vi "Concatenate_Blocks.vi"() -> (5 "Plug in titles":string[](array[string]), 7 "Plug in values":string[](array[string]))   [LabVIEW 2010]
uses:
  Controls/Instrument_Array.ctl
  Controls/Post_Process.ctl
  Controls/Graph_Type.ctl
  Globals/Meas_global.vi
  Acquisition/PWA/PWAtasksGLOBAL.vi
  Globals/Plug_in_data_global.vi
  <vilib>/Analysis/NI_AALBase.lvlib
  <vilib>/Analysis/NI_AALPro.lvlib
panel:
  in  "Inst Array":T1
  in  "Show Smooth":bool=TRUE
  in  "Save Spectra?":bool
  in  "Desired number of samples per block":i32=4096
  in  "Calculate Spectra and Histogram?":bool
  out "Spectra":cluster{dbl, dbl, "Spectrum output array":dbl[]}(graph)
  in  "Averaging samples":i32=5 min=1 max=1000
  out "XY Graph":cluster{"Axis":dbl[], "Histogram":i32[]}(graph)
  in  "Specta Index":i32
  out "Waveform Graph":dbl[][](graph)
  in  "Channels to Plot":i32[](array[ring])=[0] items=["FF (C)", "Save Nothing"]
  # "Run this VI to update the channel names"
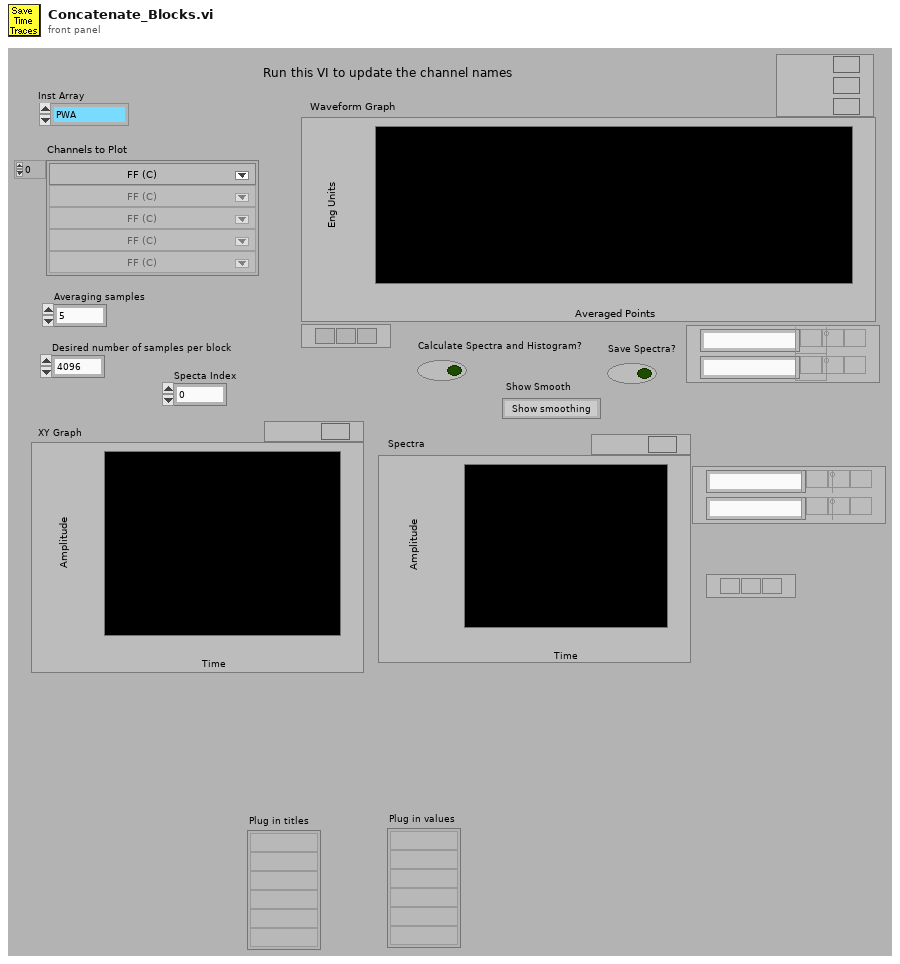
[diagram p1: front panel]
types:
  T1 = typedef "Instrument_Array.ctl" = enum16{"PWA", "LDA", "Analogue"}
  T2 = typedef "Analysis_info_cluster.ctl" = cluster{"Colour":u32, "Inst type":T3, "Inst name":string, "Symbol":string, "Code name":string, "Extra Info":string, "Inst Array":T1, "Index":i32, "Voltage Index":i32, "Extra Titles":string[], "Extra Values":string[]}
  T3 = typedef "Inst_type.ctl" = enum16{"Propeller anemometer", "Raw voltage", "Pressure Transducer", "Pitot-static tube", "Preston tube", "Hot wire", "Cross wire 1", "Cross wire 2", "Generic Linear", "Generic Polynomial", "Generic BackPoly", "Fast FID", "Thermocouple", "Cold wire", "Pulsed Wire", "LDA Vel", "LDA Tran time", "LDA Arr time"}
  T4 = typedef "Post_Process.ctl" = enum16{"Take New Data", "Post Process Raw Data File"}
  T5 = typedef "Graph_Type.ctl" = enum16{"Show no graph", "Voltage trace", "Velocity trace", "Vel histogram", "Spectrum", "f.E(f) v Log f", "Auto-Corr"}
  T6 = cluster{"Plot 1":u16, "Plot 2":u16, "Save graph":u16, "Plot Type":T5}
  T7 = cluster{dbl, dbl, "Spectrum output array":dbl[]}[]
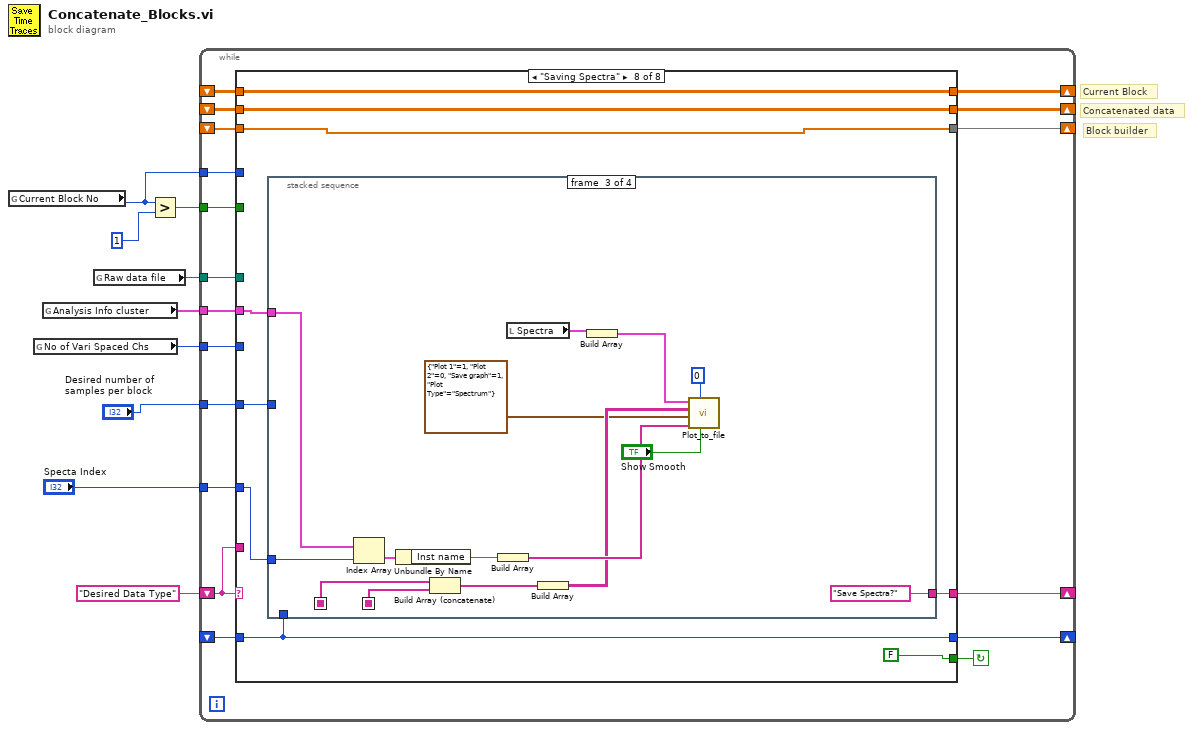
[diagram p0: block diagram]
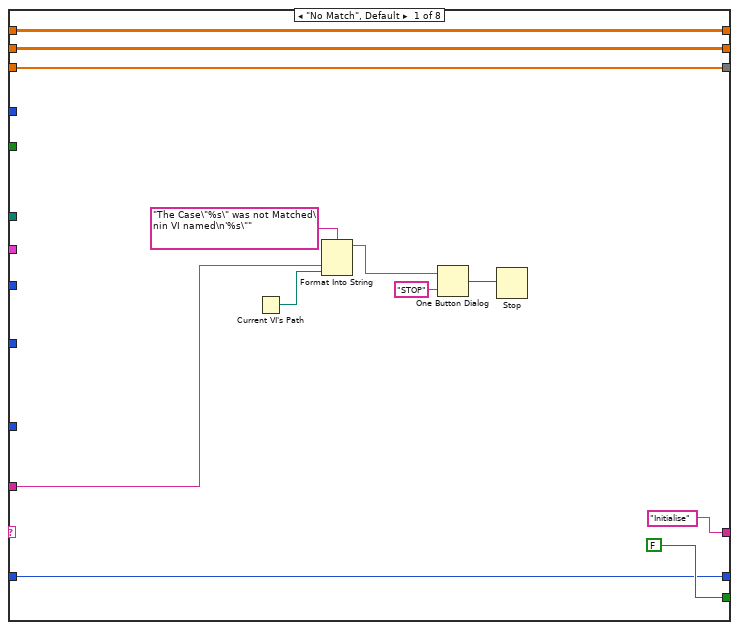
[diagram p2: hidden frame]
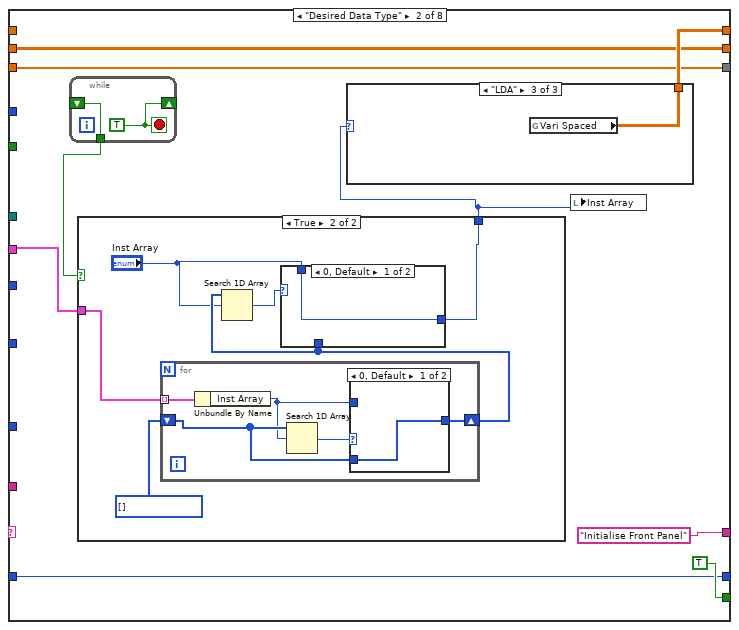
[diagram p3: hidden frame]
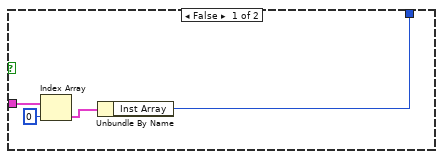
[diagram p4: hidden frame]
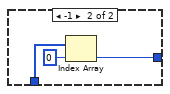
[diagram p5: hidden frame]
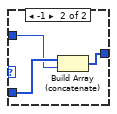
[diagram p6: hidden frame]
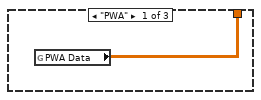
[diagram p7: hidden frame]
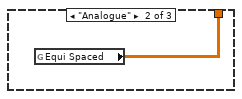
[diagram p8: hidden frame]
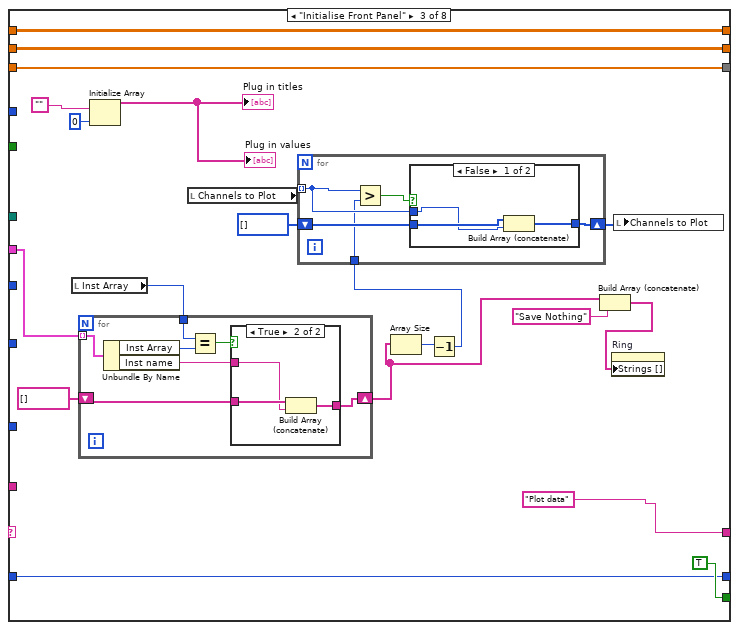
[diagram p9: hidden frame]
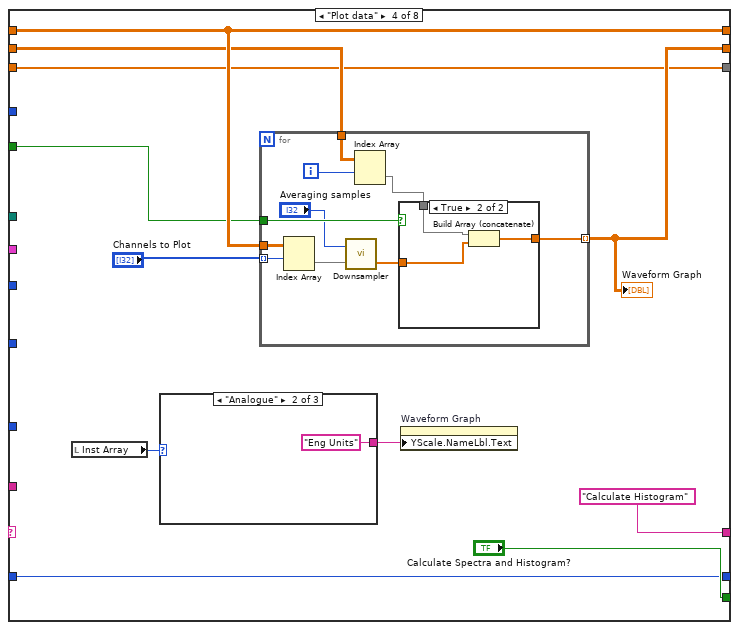
[diagram p12: hidden frame]
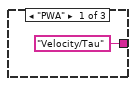
[diagram p13: hidden frame]
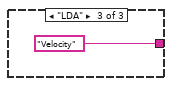
[diagram p14: hidden frame]
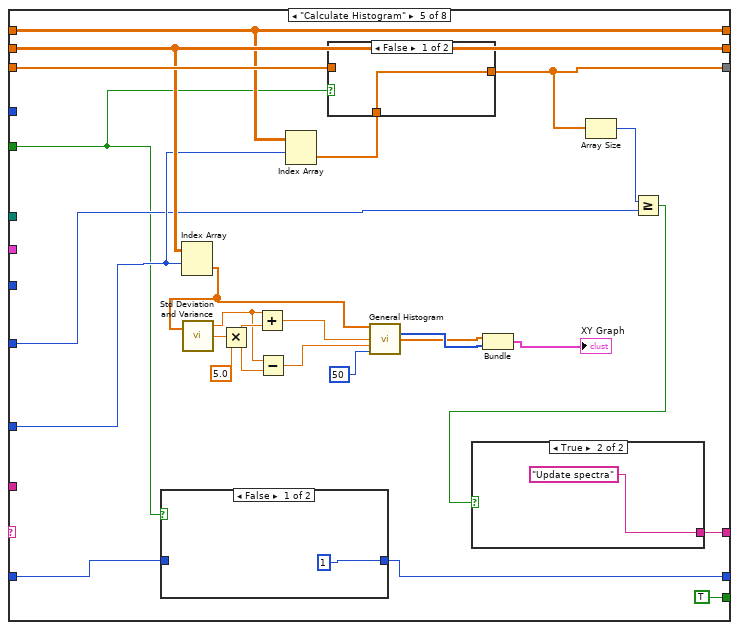
[diagram p16: hidden frame]
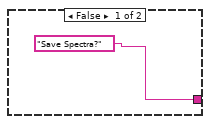
[diagram p18: hidden frame]
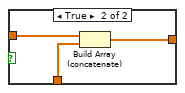
[diagram p19: hidden frame]
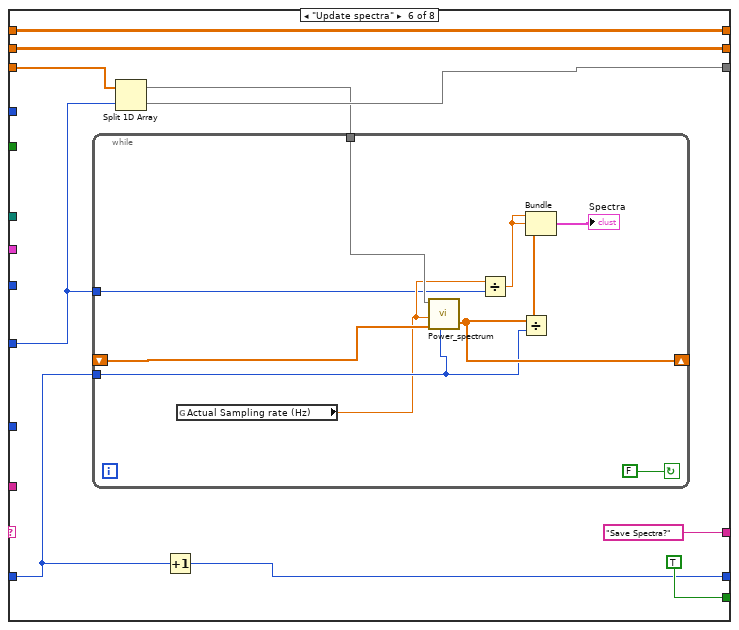
[diagram p20: hidden frame]
diagram:
  # "Block builder"
  # "Concatenated data"
  # "Current Block"
  n1 = global read "Meas_global.vi" "Current Block No"() -> (w6:i32)
  n2 = global read "Meas_global.vi" "No of Vari Spaced Chs"() -> (w4:i32)
  n3 = global read "Meas_global.vi" "Analysis Info cluster"() -> (w5:T2[])
  n4 = global read "Meas_global.vi" "Raw data file"() -> (w8:path)
  n5 = Greater?(x=w6, y=1) -> (0:w3:bool)
  n6 = while {
    shift-left: "Desired Data Type" -> [w25]
    shift-right: [w26] -> _
    tunnel: w8 -> [w24]
    tunnel: w3 -> [w23]
    tunnel: w6 -> [w22]
    tunnel: w5 -> [w21]
    tunnel: w4 -> [w20]
    shift-right: [w19] -> _
    shift-left: _ -> [w18]
    shift-right: [w16] -> _
    shift-left: _ -> [w17]
    shift-right: [w14] -> _
    shift-left: _ -> [w15]
    tunnel: "Desired number of samples per block" -> [w13]
    tunnel: "Specta Index" -> [w12]
    shift-right: [w11] -> _
    shift-left: _ -> [w10]
    stop <- w27 continue-if-true
    n7 = case shown="\"Saving Spectra\"" w25 {
      tunnel: [FALSE TRUE TRUE "Calculate Spectra and Histogram?" TRUE ("Calculate Spectra and Histogram?") TRUE ("Calculate Spectra and Histogram?") w199 FALSE ("Calculate Spectra and Histogram?")] -> w27
      tunnel: ["Initialise" "Initialise Front Panel" "Plot data" "Calculate Histogram" ("t") w149 "Save Spectra?" "Saving Spectra" w212] -> w26
      tunnel: w25 -> [w34 _ _ _ _ _ _ _]
      tunnel: w24 -> [_ _ _ _ _ _ _ _]
      tunnel: w23 -> [_ _ _ w125 w148 _ _ _]
      tunnel: w22 -> [_ _ _ _ _ _ _ _]
      tunnel: w21 -> [_ w41 w80 _ _ _ _ w210]
      tunnel: w20 -> [_ _ _ _ _ _ _ _]
      tunnel: [w31 w46 w86 w127 w157 w186 w204 w213] -> w19
      tunnel: w18 -> [w31 _ w86 w127 w157 w186 w204 w213]
      tunnel: w17 -> [w30 w45 w85 w126 w158 w187 w205 w214]
      tunnel: [w30 w45 w85 w123 w158 w187 w205 w214] -> w16
      tunnel: w15 -> [w29 w44 w82 w120 w159 w185 w202 w211]
      tunnel: [w29 w44 w82 w120 w155 w184 w202 w211] -> w14
      tunnel: w13 -> [_ _ _ _ w151 w180 _ w207]
      tunnel: w12 -> [_ _ _ _ w153 _ _ w209]
      tunnel: [w28 w43 w81 w119 w147 w178 w198 w206] -> w11
      tunnel: w10 -> [w28 w43 w81 w119 w146 w179 w198 w206]
      frame "No Match", Default {
        n8 = Current VI's Path() -> (path=w33:path)
        n9 = Format Into String(format string="The Case\"%s\" was not Matched\nin VI named\n'%s\"" ("Format String"), w34, w33) -> (resulting string=w37:string)  [unwired: 2 in, 1 out]
        n10 = One Button Dialog(message=w37, button name ("OK")="STOP") -> (true=w35:bool)
        n11 = Stop(stop? (T)=w35) -> ()
      }
      frame "Desired Data Type" {
        n12 = while {
          shift-right: [w73] -> _
          shift-left: _ -> [w72]
          tunnel: [w72] -> w42
          stop <- w73 stop-if-true
          w73 = TRUE
        }
        n13 = case shown="True" w42 {
          tunnel: w41 -> [w52 w58]
          tunnel: [w49 w54] -> w40
          frame False {
            n14 = Index Array(array=w52, index=0) -> (element=w50:T2)
            n15 = Unbundle By Name(w50) -> ("Inst Array"=w49:T1)
          }
          frame True {
            w57 = T1[] [] items=["PWA", "LDA", "Analogue"]
            n16 = for {
              tunnel: w58 -> [w67] mode=indexing
              shift-right: [w63] -> w55
              shift-left: w57 -> [w65]
              n17 = Unbundle By Name(w67) -> ("Inst Array"=w64:T1)
              n18 = Search 1D Array(1D array=w65, element=w64) -> (index of element=w66:i32)  [unwired: 1 out]
              n19 = case shown="0, Default" w66 {
                tunnel: w65 -> [w68 w71]
                tunnel: w64 -> [_ w70]
                tunnel: [w68 w69] -> w63
                frame 0, Default {
                }
                frame -1 {
                  n20 = Build Array (concatenate)(w71, w70) -> (w69:T1[])
                }
              }
            }
            n21 = Search 1D Array(1D array=w55, element="Inst Array") -> (index of element=w56:i32)  [unwired: 1 out]
            n22 = case shown="0, Default" w56 {
              tunnel: w55 -> [_ w61]
              tunnel: [w59 w60] -> w54
              tunnel: "Inst Array" -> [w59 _]
              frame 0, Default {
              }
              frame -1 {
                n23 = Index Array(array=w61, index=0) -> (element=w60:T1)
              }
            }
          }
        }
        n24 = case shown="\"LDA\"" w40 {
          tunnel: [w74 w75 w76] -> w46
          frame "PWA" {
            n25 = global read "PWAtasksGLOBAL.vi" "PWA Data"() -> (w74:dbl[][])
          }
          frame "Analogue" {
            n26 = global read "Plug_in_data_global.vi" "Equi Spaced"() -> (w75:dbl[][])
          }
          frame "LDA" {
            n27 = global read "Plug_in_data_global.vi" "Vari Spaced"() -> (w76:dbl[][])
          }
        }
        n28 = local write "Inst Array"(w40) -> ()
      }
      frame "Initialise Front Panel" {
        n29 = local read "Inst Array"() -> (w79:T1)
        n30 = for {
          tunnel: w79 -> [w102]
          tunnel: w80 -> [w101] mode=indexing
          shift-right: [w98] -> w78
          shift-left: string[] [] -> [w99]
          n31 = Unbundle By Name(w101) -> ("Inst Array"=w103:T1, "Inst name"=w97:string)
          n32 = Equal?(x=w102, y=w103) -> (x = y?=w100:bool)
          n33 = case shown="True" w100 {
            tunnel: w99 -> [w104 w107]
            tunnel: [w104 w106] -> w98
            tunnel: w97 -> [_ w105]
            frame False {
            }
            frame True {
              n34 = Build Array (concatenate)(w107, w105) -> (w106:string[])
            }
          }
        }
        n35 = Initialize Array("", 0) -> (→"Plug in values" →"Plug in titles":string[])
        n36 = local read "Channels to Plot"() -> (w93:i32[])
        n37 = Array Size(array=w78) -> (size(s)=w88:i32)
        n38 = Decrement(x=w88) -> (x-1=w87:i32)
        n39 = for {
          tunnel: w93 -> [w109] mode=indexing
          shift-right: [w110] -> w91
          shift-left: i32[] [] -> [w111]
          tunnel: w87 -> [w108]
          n40 = Greater?(x=w109, y=w108) -> (0:w112:bool)
          n41 = case shown="False" w112 {
            tunnel: w111 -> [w115 w116]
            tunnel: [w114 w116] -> w110
            tunnel: w109 -> [w113 _]
            frame False {
              n42 = Build Array (concatenate)(w115, w113) -> (w114:i32[])
            }
            frame True {
            }
          }
        }
        n43 = Build Array (concatenate)(w78, "Save Nothing") -> (w89:string[])
        n44 = property on="Ring" class="Ring (strict)"("Strings []"=w89) -> ()  [unwired: 2 in, 2 out]
        n45 = local write "Channels to Plot"(w91) -> ()
      }
      frame "Plot data" {
        n46 = local read "Inst Array"() -> (w118:T1)
        n47 = case shown="\"Analogue\"" w118 {
          tunnel: ["Velocity/Tau" "Eng Units" "Velocity"] -> w117
          frame "PWA" {
          }
          frame "Analogue" {
          }
          frame "LDA" {
          }
        }
        n48 = for {
          tunnel: w127 -> [w140]
          tunnel: "Channels to Plot" -> [w139] mode=indexing
          tunnel: w126 -> [w136]
          tunnel: [w137] -> w123 mode=indexing
          tunnel: w125 -> [w138]
          i -> [w135]
          n49 = Index Array(array=w140, index (row)=w139) -> (element=w133:dbl[])  [unwired: 1 in]
          n50 = call "Downsampler.vi"("Input Array"=w133, "Averaging samples"="Averaging samples") -> ("Downsampled Array"=w132:dbl[])  [unwired: 1 out]
          n51 = Index Array(array=w136, index (row)=w135) -> (element=w134:dbl[])  [unwired: 1 in]
          n52 = case shown="True" w138 {
            tunnel: w134 -> [_ w144]
            tunnel: w132 -> [w141 w143]
            tunnel: [w141 w142] -> w137
            frame False {
            }
            frame True {
              n53 = Build Array (concatenate)(w144, w143) -> (w142:dbl[])
            }
          }
        }
        "Waveform Graph" <- w123
        n54 = property on="Waveform Graph" class="WFGraph (strict)"("YScale.NameLbl.Text"=w117) -> ()  [unwired: 2 in, 2 out]
      }
      frame "Calculate Histogram" {
        n55 = case shown="False" w148 {
          tunnel: [1 w171] -> w147
          tunnel: w146 -> [_ w171]
          frame False {
          }
          frame True {
          }
        }
        n56 = Index Array(array=w158, index (row)=w153) -> (element=w145:dbl[])  [unwired: 1 in]
        n57 = call <vilib>:"Std Deviation and Variance.vi"("X"=w145) -> ("mean"=w162:dbl, "standard deviation"=w163:dbl)  [unwired: 1 in, 1 out]
        n58 = Multiply(x=w163, y=5.0) -> (x*y=w165:dbl)
        n59 = Add(x=w162, y=w165) -> (x+y=w161:dbl)
        n60 = Subtract(x=w162, y=w165) -> (x-y=w160:dbl)
        n61 = Index Array(array=w157, index (row)=w153) -> (element=w156:dbl[])  [unwired: 1 in]
        n62 = case shown="False" w148 {
          tunnel: w159 -> [_ w177]
          tunnel: [w174 w176] -> w155
          tunnel: w156 -> [w174 w175]
          frame False {
          }
          frame True {
            n63 = Build Array (concatenate)(w177, w175) -> (w176:dbl[])
          }
        }
        n64 = call <vilib>:"General Histogram.vi"("X"=w145, "max"=w161, "min"=w160, "# bins"=50) -> ("Histogram"=w167:i32[], "Axis"=w166:dbl[])  [unwired: 2 in, 8 out]
        n65 = Bundle("Axis"=w166, "Histogram"=w167) -> (→"XY Graph":cluster{"Axis":dbl[], "Histogram":i32[]})  [unwired: 1 out]
        n66 = Array Size(array=w155) -> (size(s)=w154:i32)
        n67 = Greater Or Equal?(x=w154, y=w151) -> (x >= y?=w150:bool)
        n68 = case shown="True" w150 {
          tunnel: ["Save Spectra?" ("f") "Update spectra"] -> w149
          frame False {
          }
          frame True {
          }
        }
      }
      frame "Update spectra" {
        n69 = Split 1D Array(array=w185, index=w180) -> (first subarray=w181:dbl[], second subarray=w184:dbl[])
        n70 = while {
          shift-left: _ -> [w194]
          shift-right: [w197] -> _
          tunnel: w181 -> [w195]
          tunnel: w179 -> [w193]
          tunnel: w180 -> [w191]
          stop <- FALSE continue-if-true
          n71 = global read "Meas_global.vi" "Actual Sampling rate (Hz)"() -> (w192:dbl)
          n72 = call "Power_spectrum.vi"("U"=w195, "Sampling frequency"=w192, "Spectrum input array"=w194, "Block No"=w193) -> ("Spectrum output array"=w197:dbl[])  [unwired: 1 in, 1 out]
          n73 = Divide(x=w192, y=w191) -> (x/y=w189:dbl)
          n74 = Divide(x=w197, y=w193) -> (x/y=w188:dbl[])
          n75 = Bundle(w189, w189, w188) -> (→"Spectra":cluster{dbl, dbl, dbl[]})  [unwired: 1 out]
        }
        n76 = Increment(x=w179) -> (x+1=w178:i32)
      }
      frame "Save Spectra?" {
        n77 = global read "Meas_global.vi" "Processing last block?"() -> (w200:bool)
        n78 = And(x=w200, y="Save Spectra?") -> (x .and. y?=w199:bool)
      }
      frame "Saving Spectra" {
        n79 = stacked-sequence {
          seq-local: [w218 _ _ _] -> [_ _ w251 _]
          seq-local: [_ w238 _ _] -> [_ _ w250 _]
          tunnel: [_ _ "Save Spectra?" _] -> w212
          tunnel: w210 -> [_ _ w257 _]
          tunnel: w209 -> [_ _ w256 _]
          tunnel: w207 -> [w216 _ _ _]
          tunnel: w206 -> [_ w236 _ _]
          frame #0 {
            n80 = global read "Meas_global.vi" "Post Process"() -> (w220:T4)
            n81 = Equal?(x=w220, y=Post_Process."Take New Data" ("Post Process")) -> (x = y?=w221:bool)
            n82 = case shown="False" w221 {
              tunnel: [w229 w233] -> w222
              frame False {
                n83 = global read "Meas_global.vi" "Pre Setup String"() -> (w230:string)
                n84 = call "Get_value_from_string.vi"("Input string"=w230, "Variable name"="Seconds since 1/1/04") -> ("Value"=w229:dbl)  [unwired: 1 in, 1 out]
              }
              frame True {
                n85 = Get Date/Time In Seconds() -> (seconds since 1Jan1904=w232:timestamp)
                n86 = To Double Precision Float(number=w232) -> (double precision float=w233:dbl)
              }
            }
            n87 = To Unsigned Long Integer(number=w222) -> (unsigned 32bit integer=w226:u32)
            n88 = Get Date/Time String(date format (0)=enum16{"short", "long", "abbreviated"}."abbreviated", seconds (now)=w226) -> (date string=w224:string, time string=w225:string)  [unwired: 1 out]
            n89 = Number To Decimal String(number=w226) -> (decimal integer string=w227:string)  [unwired: 1 out]
            n90 = Number To Decimal String(number=w216) -> (decimal integer string=w215:string)  [unwired: 1 out]
            n91 = Build Array("Time of meas", w224, w225, w227, "Block Length" ("element"), w215) -> (w218:string[])
          }
          frame #1 {
            n92 = global read "Meas_global.vi" "Actual Sampling rate (Hz)"() -> (w239:dbl)
            n93 = Decrement(x=w236) -> (x-1=w235:i32)
            n94 = global read "Meas_global.vi" "Raw data file"() -> (w245:path)
            n95 = global read "Meas_global.vi" "Comments"() -> (w244:string)
            n96 = Number To Decimal String(number=w235) -> (decimal integer string=w234:string)  [unwired: 1 out]
            n97 = Number To Fractional String(number=w239, precision (6)=i16 2) -> (F-format string=w242:string)  [unwired: 2 out]
            n98 = call "Path_2_String.vi"("Real Path"=w245) -> ("Path String"=w246:string)
            n99 = Build Array("No of Blocks", w234, "Frequency (Hz)", w242, "Raw Data file", w246, w244) -> (w238:string[])
          }
          frame #2 {
            n100 = Index Array(array=w257, index=w256) -> (element=w255:T2)
            n101 = Unbundle By Name(w255) -> ("Inst name"=w254:string)
            n102 = Build Array (concatenate)(w251, w250) -> (w249:string[])
            n103 = Build Array(w254) -> (w253:string[])
            n104 = local read "Spectra"() -> (w260:cluster{dbl, dbl, "Spectrum output array":dbl[]})
            n105 = Build Array(w249) -> (w248:string[][])
            n106 = Build Array(w260) -> (w259:T7)
            n107 = call "Plot_to_file.vi"("Show Smooth"="Show Smooth", "Start trace No"=0, "Trace names"=w253, "Graph"=T6 {"Plot 1"=1, "Plot 2"=0, "Save graph"=1, "Plot Type"=enum."Spectrum"}, "Plot file label"=w248, "Plot data"=w259) -> ()  [unwired: 6 out]
          }
          frame #3 {
            n108 = local write "Show Smooth"(FALSE ("Show Smooth")) -> ()
          }
        }
      }
    }
  }
